vi "Configure Systems.vi"() -> ()   [LabVIEW 2009, in "POLARIS BME DG.lvlib" / "BME_DG_System.lvclass"]
doc: "Use this VI for creating a configuration file.\n\nUSAGE\n\n1. Detect all DGs. This action deaktivates all DGs. Make sure you plant will not be damage by this action.\n2. Create one or more systems by enter a systemname\n3. Add at leas one master and his slaves appropriate to Your HW configuration to system\n\n4. Switch to tab Define Cards. \n5. The array index is equal DGNr of DG. Name Your Cards an configure it\n6. Enter logical names for card channels\n\n7. Switch to tab Define Channels \n8. You can start by coping channel names from the card configuration\n9. Configure Your channels.\n\nTips:\nIf \"Error?\" is true some trouble inside delay formulas is detected. Pleace throw a glance into tab \"Check\", problem channels array may give You a hint.\nThe tab contains also a tool for calculation bit masks for \"Go Signal\" in channel configiration and for MS-Bus in cards configuration.\n\n---------------\n\nauthor: Alexander Kessler, Helmholtz-Institut-Jena \nmaintainer: Alexander Kessler: alexander.kessler@uni-jena.de\n\n\nLicense Agreement for this software:\n\nCopyright (C)\nHelmholtz-Institut-Jena\nFröbelsteg 3\n07743 Jena\nGermany\n\nContact: alexander.kessler@uni-jena.de\n\nThis program is free software; you can redistribute it and/or modify it under the terms of the GNU General Public License as published by the Free Software Foundation; either version 2 of the license, or (at your option) any later version.\n\nThis program is distributed in the hope that it will be useful, but WITHOUT ANY WARRANTY; without even the implied warranty of MERCHANTABILITY or FITNESS FOR A PARTICULAR PURPOSE. See the GNU General License for more details (http://www.gnu.org)."
uses:
  BME_DG_System.lvclass
  LV-BME Interface/DetectDG.ctl
  LV-BME Interface/System DG Selection.ctl
  LV-BME Interface/BME_DG_TriggerSettings.ctl
  LV-BME Interface/ClockSource.ctl
  LV-BME Interface/SG08_Settings.ctl
  LV-BME Interface/BME_DG_V2TriggerSettings.ctl
  LV-BME Interface/MSBusSignals.ctl
  LV-BME Interface/ChnlSettings.ctl
  LV-BME Interface/Go_Done_Chnl_Settings.ctl
  LV-BME Interface/GoSignalBits.ctl
  LV-BME Interface/SG08_Chnl_Settings.ctl
  LV-BME Interface/Chnl Settings Complete.ctl
  LV-BME Interface/Card Config.ctl
  BME_DG_Chnl/BME_DG_Chnl.lvclass
  POLARIS BME DG.lvlib
panel:
  out "Error?":bool
  in  "Build System":bool
  in  "ChnlToSwap":u16(ring) items=["a", "b", "c", "d", "e", "f", "ma", "mb", "mc", "md", "me", "mf", "sa", "sb", "sc", "sd", "se", "sf"]
  in  "SwapChnlWith":bool
  in  "Card2":u16(ring) caption="Swap with" items=["Master", "Master of Slave", "Slave of Master"]
  in  "SwapCardsWith":bool
  in  "Stop search":bool=TRUE
  in  "Find Chnl":u16(ring) items=["a", "b", "c", "d", "e", "f", "ma", "mb", "mc", "md", "me", "mf", "sa", "sb", "sc", "sd", "se", "sf"]
  in  "Find Card":u16(ring) items=["Master", "Master of Slave", "Slave of Master"]
  in  "stop":bool
  in  "Tab Control":T1(tab)=enum."Check"
  in  "InstalledDGs":T2[](array[typedef])
  in  "Select System":u16(ring) items=["Einsamer Master", "Master and Servant"]
  in  "Systems":T3[](array[typedef])
  in  "Selected DG":u16(ring) items=["0", "1", "2"]
  in  "Add":bool
  in  "Remove":bool
  in  "Empty Systems":bool
  in  "DetectDGs":bool
  in  "Card Config":T9(array[cluster]) {"Advanced Settings"."Trigger on MS Bus" format="%04x" items=["Local Primary0x1"=1, "Local Secondary0x2"=2, "Local Force 0x4"=4, "Resynchronize 0x8"=8, "StepBackOnBus 0x10"=16, "StartOnBus 0x20"=32, "InhibitOnBus 0x40"=64, "LoadDataOnBus 0x80"=128]; "Advanced Settings"."Force Trigger (µs)" min=0.0 format="%.6f"; "SG08_Settings"."StepBackTime (µs)" min=0.0 format="%.6f"; "SG08_Settings"."Gate Delay (µs)" format="%.3f"; "SG08_Settings"."Gate Level" min=-2.5 max=2.5 format="%.3g"; "Base Settings"."Gate Divider" min=1 max=1000000; "Base Settings"."Clock Source" items=["Internal Oscillator"=1, "External Trigger"=2, "Trigger-> Oscillator"=3, "MasterSlave Bus"=4]; "Base Settings"."Inhibit(µs)" format="%#_11g"}
  in  "Copy Chnl\n Names":bool=TRUE
  in  "Chnls":T14(array[cluster]) {"ChnParameter"."Delay (µs)" min=0.0 max=100000000.0 format="%.4f"; "G08_Chnl_Settings"."Pulse Width (µs)" min=0.0 max=8947840.0 format="%#.6f"; "Go and Done Signal"."Done Signal" format="%04x" items=["Local Primary"=1, "Local Secondary"=2, "Local Force"=4, "Master Primary"=16]; "Go and Done Signal"."Go Signal" format="%04x" items=["Local Primary0x1"=1, "Local Secondary0x2"=2, "Local Force 0x4"=4, "Resynchronize 0x8"=8, "Master Prim. 0x10"=16, "Master Sec. 0x20"=32, "Master Force  0x40"=64, "System Clock 0x80"=128, "Delay Clock 0x100"=256, "Inhibit Local 0x200"=512, "Start Local 0x400"=1024, "Start Bus 0x800"=2048, "Step Back Local 0x1000"=4096, "Step Back Bus 0x2000"=8192, "RunCircle 0x4000"=16384, "SyncReload 0x8000"=32768, "From E 0x10000"=65536, "From F 0x20000"=131072, "From Bus 0x40000"=262144]}
  in  "MS Signals Mask":u32 caption="Mask" format="%.0x"
  in  "MS Signals Bits to Mask":T8[](array[typedef]) format="%04x" items=["Local Primary0x1"=1, "Local Secondary0x2"=2, "Local Force 0x4"=4, "Resynchronize 0x8"=8, "StepBackOnBus 0x10"=16, "StartOnBus 0x20"=32, "InhibitOnBus 0x40"=64, "LoadDataOnBus 0x80"=128]
  in  "GoSignal Bits to Mask":T12[](array[typedef]) format="%04x" items=["Local Primary0x1"=1, "Local Secondary0x2"=2, "Local Force 0x4"=4, "Resynchronize 0x8"=8, "Master Prim. 0x10"=16, "Master Sec. 0x20"=32, "Master Force  0x40"=64, "System Clock 0x80"=128, "Delay Clock 0x100"=256, "Inhibit Local 0x200"=512, "Start Local 0x400"=1024, "Start Bus 0x800"=2048, "Step Back Local 0x1000"=4096, "Step Back Bus 0x2000"=8192, "RunCircle 0x4000"=16384, "SyncReload 0x8000"=32768, "From E 0x10000"=65536, "From F 0x20000"=131072, "From Bus 0x40000"=262144]
  in  "GoSignal Mask":u32 caption="Mask" format="%.0x"
  out "Problem Chnls out":string[](array[string])
  out "err and warnings":errorcluster[](array[cluster])
  out "Last Change":timestamp=timestamp(3422440183.453125 s since 1904-01-01)
  in  "Save":bool
  in  "Load":bool=TRUE
  in  "Config File":path
  # "DGNr"
  # "<=>"
  # "<=>"
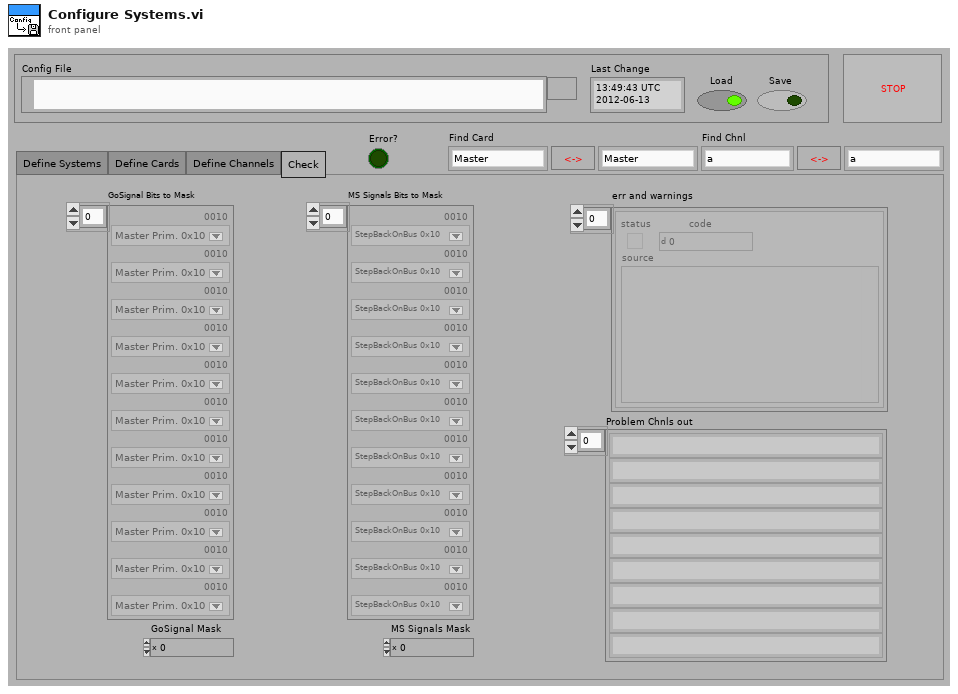
[diagram p1: front panel]
types:
  T1 = enum32{"Define Systems", "Define Cards", "Define Channels", "Check"}
  T2 = typedef "POLARIS BME DG.lvlib/DetectDG.ctl" = cluster{"DG_Number":i32, "DG_Product":i32, "Product Name":string, "Bus_Number":i32, "Slot_Number":i32, "Master":bool}
  T3 = typedef "POLARIS BME DG.lvlib/System DG Selection.ctl" = cluster{"Selected System DGs":T2[], "Name":string}
  T4 = typedef "POLARIS BME DG.lvlib/BME_DG_TriggerSettings.ctl" = cluster{"Clock Source":T5, " clock modulo":u32, "TriggerEnabled?":bool, "trigger modulo ":i32, "InputTerminated?":bool, "Inhibit(µs)":dbl, "TriggerLevel":dbl, "PresetValue":i32, "InternalTrigger?":bool, "InternalArm?":bool, "SWTrigger?":bool, "RisingEdge?":bool, "StopOnPreset?":bool, "ResetWhenDone?":bool, "Gate Divider":i32, "PositiveGate?":bool}
  T5 = typedef "POLARIS BME DG.lvlib/ClockSource.ctl" = i32
  T6 = typedef "POLARIS BME DG.lvlib/SG08_Settings.ctl" = cluster{"Gate Terminate":bool, "Gate Level":dbl, "Gate Delay (µs)":dbl, "StepBackTime (µs)":dbl, "Burst Counter":u32, "Trigger Divider":u32, "Trigger Multiplier":u32}
  T7 = typedef "POLARIS BME DG.lvlib/BME_DG_V2TriggerSettings.ctl" = cluster{"Trigger on MS Bus":T8, "Force Trigger (µs)":dbl, "Gate Type":bool, "Synchronize Gate":bool}
  T8 = typedef "POLARIS BME DG.lvlib/MSBusSignals.ctl" = u32
  T9 = cluster{"Logical Name":string, "Base Settings":T4, "SG08_Settings":T6, "Channel Names":string[], "Advanced Settings":T7}[]
  T10 = typedef "POLARIS BME DG.lvlib/ChnlSettings.ctl" = cluster{" Delay (µs)":dbl, "On?":bool, "PositiveVoltage?":bool, "50OhmTerminated? ":bool, "25OhmOutput?":bool}
  T11 = typedef "POLARIS BME DG.lvlib/Go_Done_Chnl_Settings.ctl" = cluster{"Go Signal":T12, "Done Signal":u32}
  T12 = typedef "POLARIS BME DG.lvlib/GoSignalBits.ctl" = u32
  T13 = typedef "POLARIS BME DG.lvlib/SG08_Chnl_Settings.ctl" = cluster{"Pulse Width (µs)":dbl, "Output Offset":u32, "Disconnect (E,F)":bool, "Onto MsBus (E,F)":bool, "Input Positive (E,F)":bool}
  T14 = cluster{"Channel Name":string, "ChnParameter":T10, "DelayFormula":string, "OutputModulo":i32, "Go and Done Signal":T11, "G08_Chnl_Settings":T13}[]
  T15 = typedef "POLARIS BME DG.lvlib/Chnl Settings Complete.ctl" = cluster{"Channel Name":string, "ChnParameter":T10, "DelayFormula":string, "OutputModulo":i32, "Go and Done Signal":T11, "G08_Chnl_Settings":T13}
  T16 = typedef "POLARIS BME DG.lvlib/Card Config.ctl" = cluster{"Logical Name":string, "Base Settings":T4, "SG08_Settings":T6, "Channel Names":string[], "Advanced Settings":T7}
  T17 = enum16{"open", "replace", "create", "open or create", "replace or create", "replace or create with confirmation"}
  T18 = cluster{"Logical Name":string, "Base Settings":T4, "SG08_Settings":T6, "Channel Names":string[], "Advanced Settings":T7}
  T19 = cluster{"Channel Name":string, "ChnParameter":T10, "DelayFormula":string, "OutputModulo":i32, "Go and Done Signal":T11, "G08_Chnl_Settings":T13}
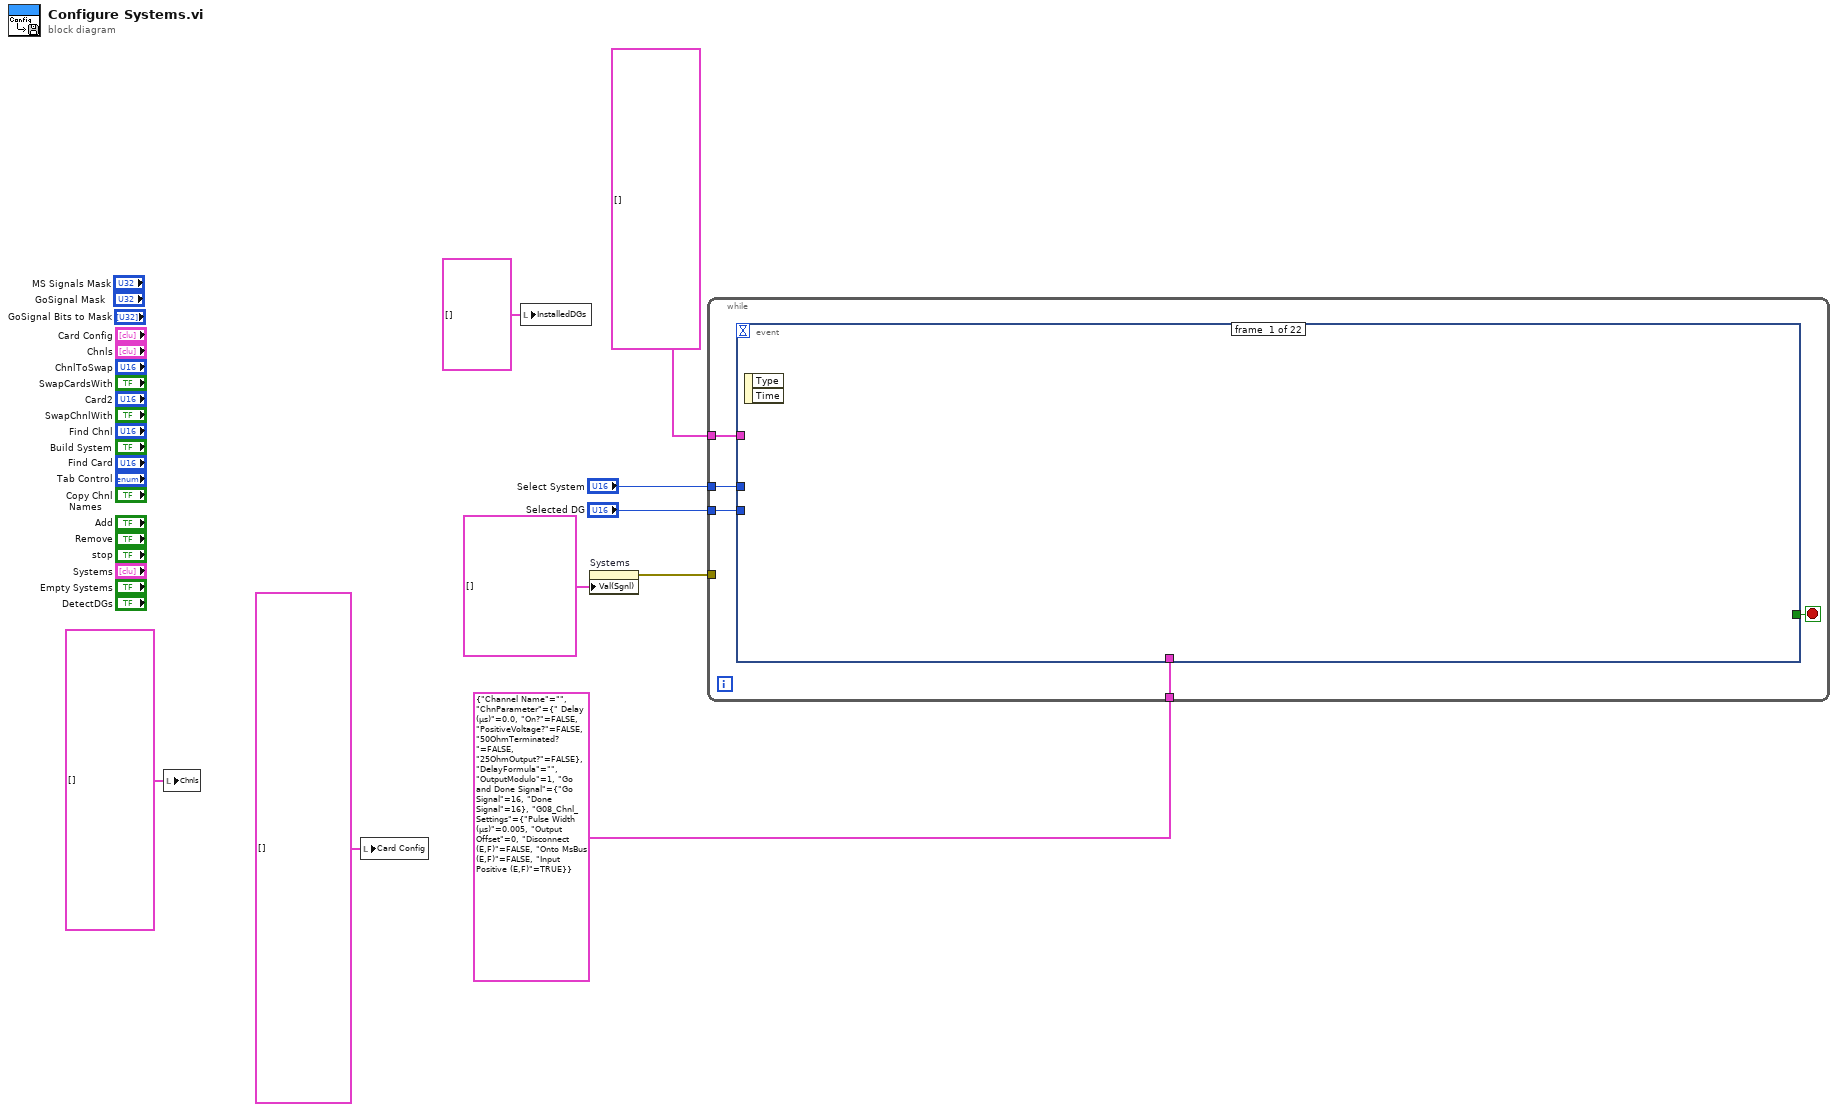
[diagram p0: block diagram]
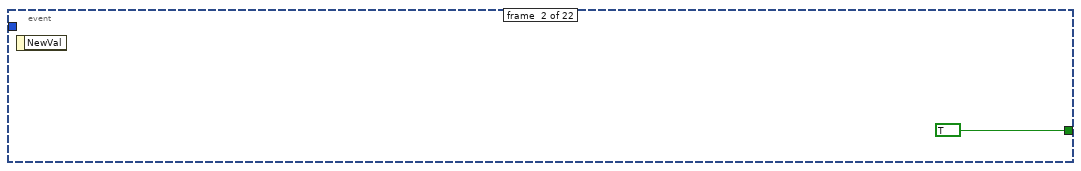
[diagram p2: hidden frame]
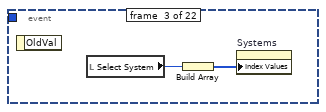
[diagram p3: hidden frame]
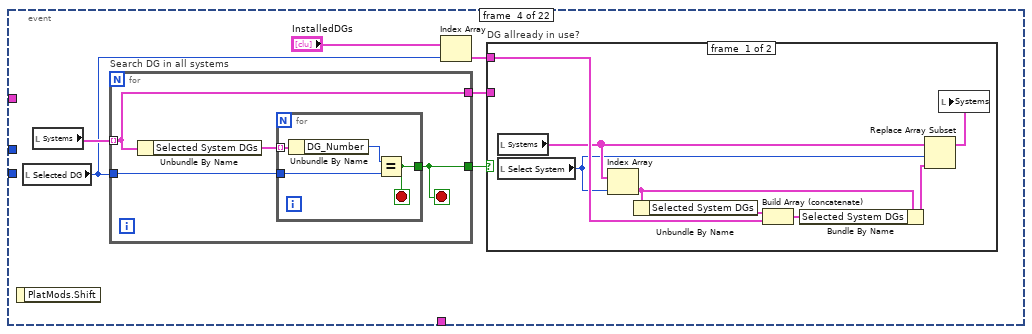
[diagram p4: hidden frame]
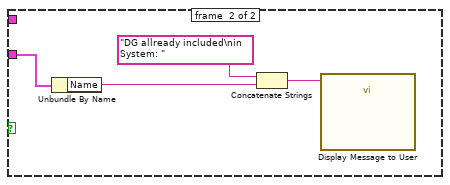
[diagram p5: hidden frame]
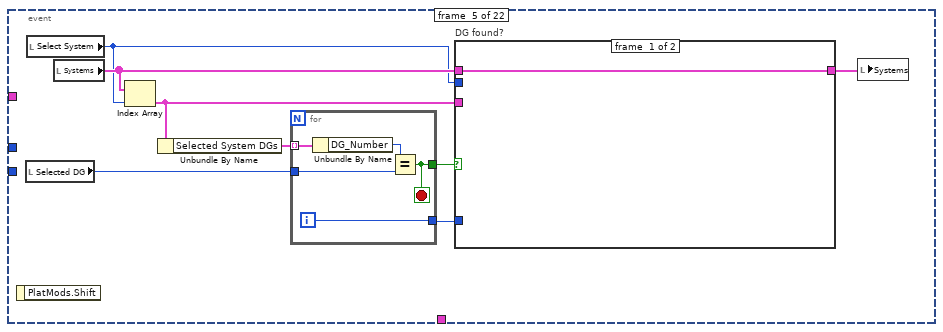
[diagram p6: hidden frame]
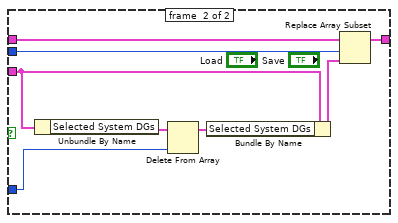
[diagram p7: hidden frame]
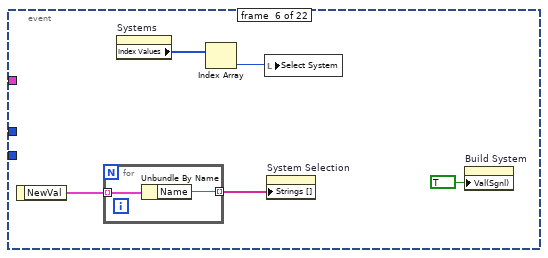
[diagram p8: hidden frame]
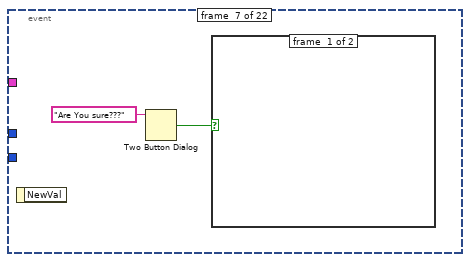
[diagram p9: hidden frame]
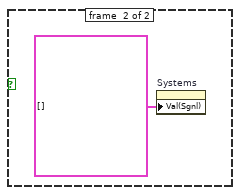
[diagram p10: hidden frame]
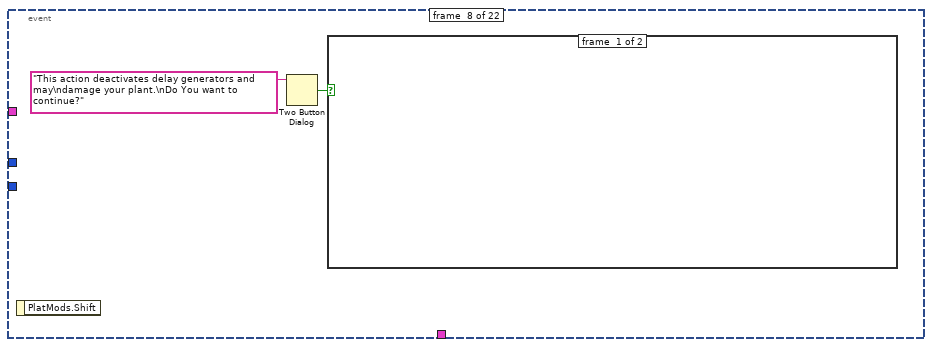
[diagram p11: hidden frame]
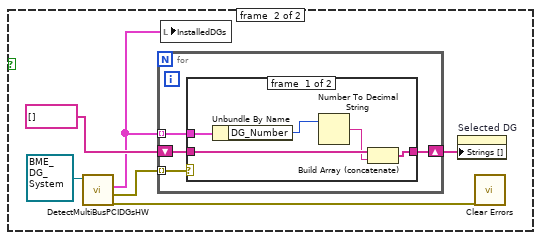
[diagram p12: hidden frame]
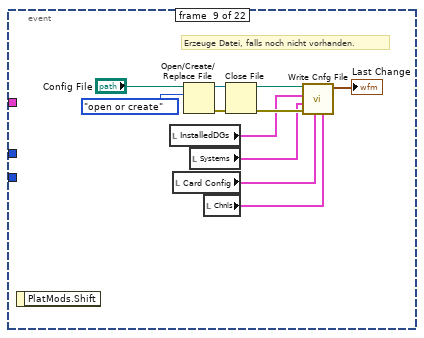
[diagram p14: hidden frame]
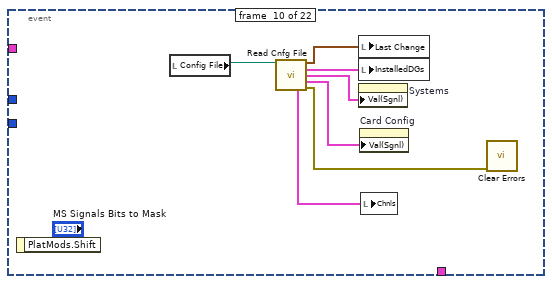
[diagram p15: hidden frame]
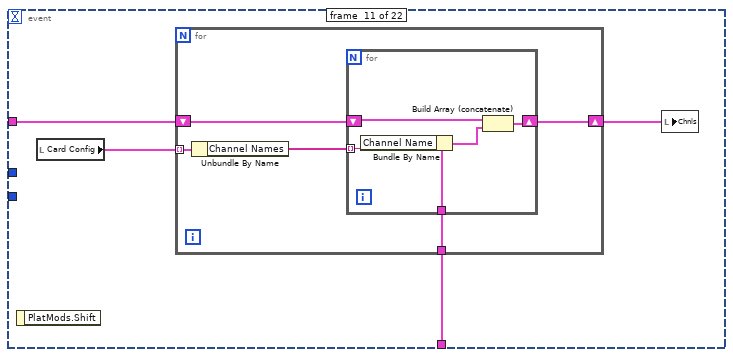
[diagram p16: hidden frame]
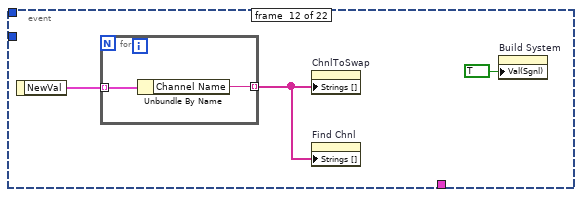
[diagram p17: hidden frame]
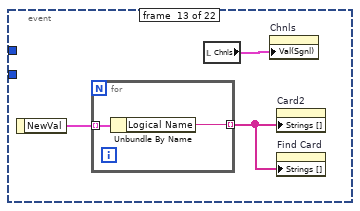
[diagram p18: hidden frame]
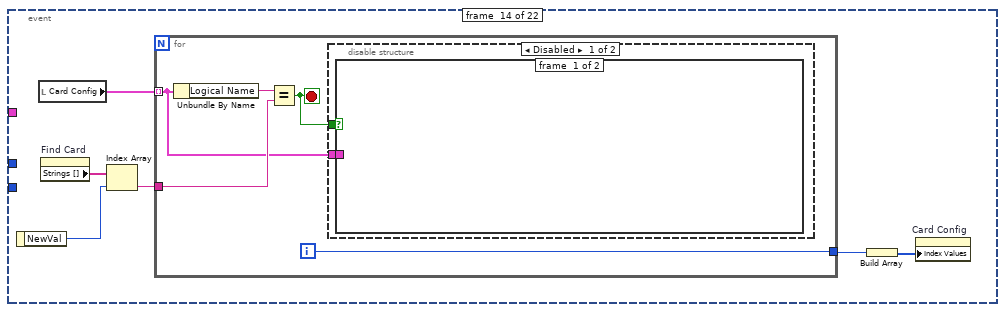
[diagram p19: hidden frame]
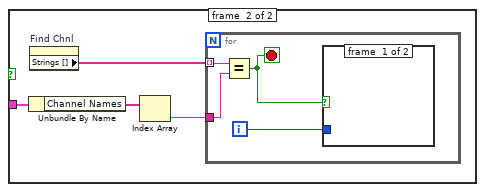
[diagram p20: hidden frame]
diagram:
  n1 = local write "Chnls"(T15[] [] ("Chnls")) -> ()
  n2 = local write "Card Config"(T16[] [] ("Card Config")) -> ()
  n3 = local write "InstalledDGs"(T2[] [] ("InstalledDGs")) -> ()
  n4 = property on="Systems" class="Arr (strict)"("Val(Sgnl)"=T3[] [] ("Value (Signaling)")) -> (error out=w6:errorcluster)  [unwired: 2 in, 1 out]
  n5 = while {
    tunnel: "Select System" -> [w13]
    tunnel: "Selected DG" -> [w12]
    tunnel: w6 -> [_]
    tunnel: T15 {"Channel Name"="", "ChnParameter"={" Delay (µs)"=0.0, "On?"=FALSE, "PositiveVoltage?"=FALSE, "50OhmTerminated? "=FALSE, "25OhmOutput?"=FALSE}, "DelayFormula"="", "OutputModulo"=1, "Go and Done Signal"={"Go Signal"=16, "Done Signal"=16}, "G08_Chnl_Settings"={"Pulse Width (µs)"=0.005, "Output Offset"=0, "Disconnect (E,F)"=FALSE, "Onto MsBus (E,F)"=FALSE, "Input Positive (E,F)"=TRUE}} ("Cluster") -> [w11]
    tunnel: T15[] [] -> [w10]
    stop <- w14 stop-if-true
    n6 = event shown="[8] \"Save\": Mouse Down;  \"Save\": Key Down" {
      selector: _ -> [_ _ _ _ _ _ _ _ _ _ _ _ _ _ _ _ _ _ _ _ _ _]
      dyn-events: _ -> [_ _ _ _ _ _ _ _ _ _ _ _ _ _ _ _ _ _ _ _ _ _]
      timeout: _ -> [_ _ _ _ _ _ _ _ _ _ _ _ _ _ _ _ _ _ _ _ _ _]
      tunnel: [_ TRUE _ _ _ _ _ _ _ _ _ _ _ _ _ _ _ _ _ _ _ _] -> w14
      tunnel: w13 -> [_ _ _ _ _ _ _ _ _ _ _ _ _ _ _ _ _ _ _ _ _ _]
      tunnel: w12 -> [_ _ _ _ _ _ _ _ _ _ _ _ _ _ _ _ _ _ _ _ _ _]
      tunnel: w11 -> [_ _ _ _ _ _ _ _ _ _ w113 _ _ _ _ _ _ _ _ _ _ _]
      tunnel: w10 -> [_ _ _ _ _ _ _ _ _ _ w112 _ _ _ _ _ _ _ _ _ _ _]
      event #0 {
        n7 = event-data() -> ()  [unwired: 1 in, 2 out]
      }
      event #1 {
        n8 = event-data() -> ()  [unwired: 1 in, 1 out]
      }
      event #2 {
        n9 = event-data() -> ()  [unwired: 1 in, 1 out]
        n10 = local read "Select System"() -> (w17:u16)
        n11 = Build Array(w17) -> (w16:u16[])
        n12 = property on="Systems" class="Arr (strict)"("Index Values"=w16) -> ()  [unwired: 2 in, 2 out]
      }
      event #3 {
        n13 = event-data() -> ()  [unwired: 1 in, 1 out]
        n14 = local read "Selected DG"() -> (w20:u16)
        n15 = local read "Systems"() -> (w23:T3[])
        n16 = for "Search DG in all systems" {
          tunnel: w23 -> [w36] mode=indexing
          tunnel: w20 -> [w38]
          tunnel: [w36] -> w21
          tunnel: [w37] -> w22
          stop <- w37 stop-if-true
          n17 = Unbundle By Name(w36) -> ("Selected System DGs"=w39:T2[])
          n18 = for {
            tunnel: w39 -> [w43] mode=indexing
            tunnel: w38 -> [w42]
            tunnel: [w40] -> w37
            stop <- w40 stop-if-true
            n19 = Unbundle By Name(w43) -> ("DG_Number"=w41:i32)
            n20 = Equal?(x=w41, y=w42) -> (x = y?=w40:bool)
          }
        }
        n21 = Index Array(array="InstalledDGs", index=w20) -> (element=w19:T2)
        n22 = case "DG allready in use?" shown="False" w22 {
          tunnel: w21 -> [_ w35]
          tunnel: w19 -> [w29 _]
          frame #0 {
            n23 = local read "Systems"() -> (w26:T3[])
            n24 = local read "Select System"() -> (w25:u16)
            n25 = Index Array(array=w26, index=w25) -> (element=w24:T3)
            n26 = Unbundle By Name(w24) -> ("Selected System DGs"=w31:T2[])
            n27 = Build Array (concatenate)(w31, w29) -> (w30:T2[])
            n28 = Bundle By Name(cluster=w24, "Selected System DGs"=w30) -> (w27:T3)
            n29 = Replace Array Subset(array=w26, new element=w27, index=w25) -> (w28:T3[])
            n30 = local write "Systems"(w28) -> ()
          }
          frame #1 {
            n31 = Unbundle By Name(w35) -> ("Name"=w32:string)
            n32 = Concatenate Strings("DG allready included\nin System: " ("string"), w32) -> (w34:string)
            n33 = call "Display Message to User"("Message"=w34) -> ()  [unwired: 9 in, 2 out]
          }
        }
      }
      event #4 {
        n34 = event-data() -> ()  [unwired: 1 in, 1 out]
        n35 = local read "Selected DG"() -> (w47:u16)
        n36 = local read "Select System"() -> (w44:u16)
        n37 = local read "Systems"() -> (w48:T3[])
        n38 = Index Array(array=w48, index=w44) -> (element=w45:T3)
        n39 = Unbundle By Name(w45) -> ("Selected System DGs"=w46:T2[])
        n40 = for {
          tunnel: w46 -> [w52] mode=indexing
          tunnel: w47 -> [w56]
          tunnel: [w55] -> w51
          tunnel: [w54] -> w50
          i -> [w54]
          stop <- w55 stop-if-true
          n41 = Unbundle By Name(w52) -> ("DG_Number"=w53:i32)
          n42 = Equal?(x=w53, y=w56) -> (x = y?=w55:bool)
        }
        n43 = case "DG found?" shown="True" w51 {
          tunnel: w50 -> [_ w62]
          tunnel: w48 -> [w57 w65]
          tunnel: [w57 w64] -> w49
          tunnel: w45 -> [_ w61]
          tunnel: w44 -> [_ w58]
          frame #0 {
          }
          frame #1 {
            n44 = Unbundle By Name(w61) -> ("Selected System DGs"=w63:T2[])
            n45 = Delete From Array(array=w63, index=w62) -> (array with subset deleted=w60:T2[])  [unwired: 1 in, 1 out]
            n46 = Bundle By Name(cluster=w61, "Selected System DGs"=w60) -> (w59:T3)
            n47 = Replace Array Subset(array=w65, new element=w59, index=w58) -> (w64:T3[])
          }
        }
        n48 = local write "Systems"(w49) -> ()
      }
      event #5 {
        n49 = event-data() -> ("NewVal"=w70:T3[])  [unwired: 1 in]
        n50 = for {
          tunnel: w70 -> [w72] mode=indexing
          tunnel: [w71] -> w69 mode=indexing
          n51 = Unbundle By Name(w72) -> ("Name"=w71:string)
        }
        n52 = property on="Systems" class="Arr (strict)"() -> ("Index Values"=w68:u32[])  [unwired: 2 in, 2 out]
        n53 = Index Array(array=w68) -> (element=w67:u32)  [unwired: 1 in]
        n54 = local write "Select System"(w67) -> ()
        n55 = property on="System Selection" class="Ring (strict)"("Strings []"=w69) -> ()  [unwired: 2 in, 2 out]
        n56 = property on="Build System" class="Bool (strict)"("Val(Sgnl)"=TRUE ("Value (Signaling)")) -> ()  [unwired: 2 in, 2 out]
      }
      event #6 {
        n57 = event-data() -> ()  [unwired: 1 in, 1 out]
        n58 = Two Button Dialog(message="Are You sure???") -> (T button?=w73:bool)  [unwired: 2 in]
        n59 = case shown="True" w73 {
          frame #0 {
          }
          frame #1 {
            n60 = property on="Systems" class="Arr (strict)"("Val(Sgnl)"=T3[] [] ("Value (Signaling)")) -> ()  [unwired: 2 in, 2 out]
          }
        }
      }
      event #7 {
        n61 = event-data() -> ()  [unwired: 1 in, 1 out]
        n62 = Two Button Dialog(message="This action deactivates delay generators and may\ndamage your plant.\nDo You want to continue?") -> (T button?=w76:bool)  [unwired: 2 in]
        n63 = case shown="True" w76 {
          frame #0 {
          }
          frame #1 {
            n64 = call "DetectMultiBusPCIDGsHW.vi"("BME_DG_System in"=refnum<class "BME_DG_System.lvclass"> refnum) -> ("error out"=w78:errorcluster, "Errors"=w81:errorcluster[], "InstalledDGs"=w79:T2[])  [unwired: 6 in, 2 out]
            n65 = for {
              tunnel: w81 -> [w84] mode=indexing
              tunnel: w79 -> [w86] mode=indexing
              shift-right: [w87] -> w82
              shift-left: string[] [] -> [w85]
              n66 = case shown="No Error" w84 {
                tunnel: [w92 w93] -> w87
                tunnel: w86 -> [w90 _]
                tunnel: w85 -> [w91 w93]
                frame #0 {
                  n67 = Unbundle By Name(w90) -> ("DG_Number"=w89:i32)
                  n68 = Number To Decimal String(number=w89) -> (decimal integer string=w88:string)  [unwired: 1 in]
                  n69 = Build Array (concatenate)(w91, w88) -> (w92:string[])
                }
                frame #1 {
                }
              }
            }
            n70 = local write "InstalledDGs"(w79) -> ()
            n71 = property on="Selected DG" class="Ring (strict)"("Strings []"=w82) -> ()  [unwired: 2 in, 2 out]
            n72 = call <vilib>:"Clear Errors.vi"("error in (no error)"=w78) -> ()  [unwired: 6 in, 1 out]
          }
        }
      }
      event #8 {
        # "Erzeuge Datei, falls noch nicht vorhanden."
        n73 = event-data() -> ()  [unwired: 1 in, 1 out]
        n74 = local read "InstalledDGs"() -> (w98:T2[])
        n75 = local read "Card Config"() -> (w96:T9)
        n76 = Open/Create/Replace File(file path (use dialog)="Config File", operation (0:open)=T17."open or create") -> (refnum out=w103:refnum<file>, error out=w102:errorcluster)  [unwired: 4 in, 1 out]
        n77 = local read "Systems"() -> (w97:T3[])
        n78 = local read "Chnls"() -> (w95:T14)
        n79 = Close File(refnum=w103, error in=w102) -> (path=w100:path, error out=w99:errorcluster)
        n80 = call "Write Cnfg File.vi"("Chnls"=w95, "Cards"=w96, "error in"=w99, "DGSystems"=w97, "InstalledDGs"=w98, "pathConfigFile"=w100) -> ("current time"=→"Last Change":timestamp)  [unwired: 4 in, 1 out]
      }
      event #9 {
        n81 = event-data() -> ()  [unwired: 1 in, 1 out]
        n82 = local read "Config File"() -> (w111:path)
        n83 = call "Read Cnfg File.vi"("Config File"=w111) -> ("Last Change"=w110:timestamp, "InstalledDGs"=w109:T2[], "DGSystems"=w108:T3[], "Cards"=w107:T16[], "Chnls"=w106:T15[], "error out"=w105:errorcluster)  [unwired: 9 in]
        n84 = local write "Last Change"(w110) -> ()
        n85 = local write "InstalledDGs"(w109) -> ()
        n86 = property on="Systems" class="Arr (strict)"("Val(Sgnl)"=w108) -> ()  [unwired: 2 in, 2 out]
        n87 = property on="Card Config" class="Arr (strict)"("Val(Sgnl)"=w107) -> ()  [unwired: 2 in, 2 out]
        n88 = local write "Chnls"(w106) -> ()
        n89 = call <vilib>:"Clear Errors.vi"("error in (no error)"=w105) -> ()  [unwired: 6 in, 1 out]
      }
      event #10 {
        n90 = event-data() -> ()  [unwired: 1 in, 1 out]
        n91 = local read "Card Config"() -> (w115:T9)
        n92 = for {
          tunnel: w115 -> [w120] mode=indexing
          shift-right: [w117] -> w114
          shift-left: w112 -> [w118]
          tunnel: w113 -> [w116]
          n93 = Unbundle By Name(w120) -> ("Channel Names"=w119:string[])
          n94 = for {
            tunnel: w119 -> [w122] mode=indexing
            shift-right: [w124] -> w117
            shift-left: w118 -> [w125]
            tunnel: w116 -> [w123]
            n95 = Bundle By Name(cluster=w123, "Channel Name"=w122) -> (w121:T15)
            n96 = Build Array (concatenate)(w125, w121) -> (w124:T15[])
          }
        }
        n97 = local write "Chnls"(w114) -> ()
      }
      event #11 {
        n98 = event-data() -> ("NewVal"=w128:T14)  [unwired: 1 in]
        n99 = for {
          tunnel: w128 -> [w129] mode=indexing
          tunnel: [w130] -> w127 mode=indexing
          n100 = Unbundle By Name(w129) -> ("Channel Name"=w130:string)
        }
        n101 = property on="ChnlToSwap" class="Ring (strict)"("Strings []"=w127) -> ()  [unwired: 2 in, 2 out]
        n102 = property on="Find Chnl" class="Ring (strict)"("Strings []"=w127) -> ()  [unwired: 2 in, 2 out]
        n103 = property on="Build System" class="Bool (strict)"("Val(Sgnl)"=TRUE ("Value (Signaling)")) -> ()  [unwired: 2 in, 2 out]
      }
      event #12 {
        n104 = event-data() -> ("NewVal"=w133:T9)  [unwired: 1 in]
        n105 = for {
          tunnel: w133 -> [w135] mode=indexing
          tunnel: [w134] -> w132 mode=indexing
          n106 = Unbundle By Name(w135) -> ("Logical Name"=w134:string)
        }
        n107 = local read "Chnls"() -> (w131:T14)
        n108 = property on="Chnls" class="Arr (strict)"("Val(Sgnl)"=w131) -> ()  [unwired: 2 in, 2 out]
        n109 = property on="Card2" class="Ring (strict)"("Strings []"=w132) -> ()  [unwired: 2 in, 2 out]
        n110 = property on="Find Card" class="Ring (strict)"("Strings []"=w132) -> ()  [unwired: 2 in, 2 out]
      }
      event #13 {
        n111 = event-data() -> ("NewVal"=w137:u16)  [unwired: 1 in]
        n112 = local read "Card Config"() -> (w139:T9)
        n113 = property on="Find Card" class="Ring (strict)"() -> ("Strings []"=w138:string[])  [unwired: 2 in, 2 out]
        n114 = Index Array(array=w138, index=w137) -> (element=w140:string)
        n115 = for {
          tunnel: w139 -> [w142] mode=indexing
          tunnel: w140 -> [w145]
          tunnel: [w144] -> w141
          i -> [w144]
          stop <- w143 stop-if-true
          n116 = Unbundle By Name(w142) -> ("Logical Name"=w146:string)
          n117 = Equal?(x=w146, y=w145) -> (x = y?=w143:bool)
          n118 = disable-structure shown="Disabled" {
            disable-tunnel: w143 -> [w148 _]
            disable-tunnel: w142 -> [w147 _]
            frame #0 {
              n119 = case shown="True" w148 {
                tunnel: w147 -> [_ w151]
                frame #0 {
                }
                frame #1 {
                  n120 = Unbundle By Name(w151) -> ("Channel Names"=w150:string[])
                  n121 = property on="Find Chnl" class="Ring (strict)"() -> ("Strings []"=w152:string[])  [unwired: 2 in, 2 out]
                  n122 = Index Array(array=w150) -> (element=w149:string)  [unwired: 1 in]
                  n123 = for {
                    tunnel: w152 -> [w156] mode=indexing
                    tunnel: w149 -> [w155]
                    i -> [w153]
                    stop <- w154 stop-if-true
                    n124 = Equal?(x=w156, y=w155) -> (x = y?=w154:bool)
                    n125 = case shown="True" w154 {
                      selector: w154 -> [_ w157]
                      tunnel: w153 -> [_ w158]
                      frame #0 {
                      }
                      frame #1 {
                        n126 = local write "Stop search"(w157) -> ()
                        n127 = property on="Find Chnl" class="Ring (strict)"("Val(Sgnl)"=w158) -> ()  [unwired: 2 in, 2 out]
                      }
                    }
                  }
                }
              }
            }
            frame #1 {
            }
          }
        }
        n128 = Build Array(w141) -> (w136:i32[])
        n129 = property on="Card Config" class="Arr (strict)"("Index Values"=w136) -> ()  [unwired: 2 in, 2 out]
      }
      event #14 {
        n130 = event-data() -> ("NewVal"=w169:u16)  [unwired: 1 in]
        n131 = local read "Card Config"() -> (w170:T9)
        n132 = property on="Find Chnl" class="Ring (strict)"() -> ("Strings []"=w168:string[])  [unwired: 2 in, 2 out]
        n133 = Index Array(array=w168, index=w169) -> (element=w163:string)
        n134 = for {
          tunnel: w170 -> [w184] mode=indexing
          tunnel: w163 -> [w182]
          tunnel: [w181] -> w167
          tunnel: [w180] -> w166
          i -> [w181]
          stop <- w180 stop-if-true
          n135 = Unbundle By Name(w184) -> ("Channel Names"=w183:string[])
          n136 = for {
            tunnel: w183 -> [w186] mode=indexing
            tunnel: w182 -> [w187]
            tunnel: [w185] -> w180
            stop <- w185 stop-if-true
            n137 = Equal?(x=w186, y=w187) -> (x = y?=w185:bool)
          }
        }
        n138 = Not(x="Stop search") -> (.not. x?=w159:bool)
        n139 = And(x=w166, y=w159) -> (x .and. y?=w161:bool)
        n140 = local read "Chnls"() -> (w165:T14)
        n141 = case shown="True" w161 {
          tunnel: w167 -> [_ w179]
          frame #0 {
            n142 = local write "Stop search"(FALSE ("Stop search")) -> ()
          }
          frame #1 {
            n143 = property on="Find Card" class="Ring (strict)"("Val(Sgnl)"=w179) -> ()  [unwired: 2 in, 2 out]
          }
        }
        n144 = for {
          tunnel: w165 -> [w177] mode=indexing
          tunnel: w163 -> [w175]
          tunnel: [w174] -> w164
          tunnel: [w173] -> w162
          i -> [w174]
          stop <- w173 stop-if-true
          n145 = Unbundle By Name(w177) -> ("Channel Name"=w176:string)
          n146 = Equal?(x=w175, y=w176) -> (x = y?=w173:bool)
        }
        n147 = case shown="True" w162 {
          tunnel: w164 -> [_ w171]
          frame #0 {
          }
          frame #1 {
            n148 = Build Array(w171) -> (w172:i32[])
            n149 = property on="Chnls" class="Arr (strict)"("Index Values"=w172) -> ()  [unwired: 2 in, 2 out]
          }
        }
      }
      event #15 {
        n150 = event-data() -> ("NewVal"=w190:T12[])  [unwired: 1 in]
        n151 = for {
          tunnel: w190 -> [w193] mode=indexing
          shift-right: [w192] -> w188
          shift-left: 0 -> [w191]
          n152 = Or(x=w191, y=w193) -> (x .or. y?=w192:T12)
        }
        n153 = local write "GoSignal Mask"(w188) -> ()
      }
      event #16 {
        n154 = event-data() -> ("NewVal"=w196:T8[])  [unwired: 1 in]
        n155 = for {
          tunnel: w196 -> [w199] mode=indexing
          shift-right: [w198] -> w194
          shift-left: 0 -> [w197]
          n156 = Or(x=w197, y=w199) -> (x .or. y?=w198:T8)
        }
        n157 = local write "MS Signals Mask"(w194) -> ()
      }
      event #17 {
        n158 = event-data() -> ("NewVal"=w200:bool)  [unwired: 1 in]
        n159 = case shown="True" w200 {
          frame #0 {
          }
          frame #1 {
            n160 = local read "Card Config"() -> (w207:T9)
            n161 = local read "Find Card"() -> (w205:u16)
            n162 = local read "Card2"() -> (w202:u16)
            n163 = Index Array(array=w207, index #1=w205, index #2=w202) -> (element #1=w203:T18, element #2=w204:T18)
            n164 = Replace Array Subset(array=w207, new element=w204, index=w205) -> (w206:T9)
            n165 = Replace Array Subset(array=w206, new element=w203, index=w202) -> (w201:T9)
            n166 = property on="Card Config" class="Arr (strict)"("Val(Sgnl)"=w201) -> ()  [unwired: 2 in, 2 out]
          }
        }
      }
      event #18 {
        n167 = event-data() -> ()  [unwired: 1 in, 2 out]
        n168 = local read "Chnls"() -> (w210:T14)
        n169 = local read "Find Chnl"() -> (w209:u16)
        n170 = local read "ChnlToSwap"() -> (w208:u16)
        n171 = Index Array(array=w210, index #1=w209, index #2=w208) -> (element #1=w212:T19, element #2=w213:T19)
        n172 = Replace Array Subset(array=w210, new element=w213, index=w209) -> (w214:T14)
        n173 = Replace Array Subset(array=w214, new element=w212, index=w208) -> (w211:T14)
        n174 = property on="Chnls" class="Arr (strict)"("Val(Sgnl)"=w211) -> ()  [unwired: 2 in, 2 out]
      }
      event #19 {
        n175 = event-data() -> ("NewVal"=w218:u32)  [unwired: 1 in]
        n176 = Number To Boolean Array(number=w218) -> (Boolean array=w217:bool[])
        n177 = for {
          tunnel: w217 -> [w222] mode=indexing
          shift-right: [w219] -> w215
          shift-left: i32[] [] ("Array") -> [w220]
          i -> [w221]
          n178 = case shown="True" w222 {
            tunnel: w221 -> [_ w227]
            tunnel: w220 -> [w223 w225]
            tunnel: [w223 w224] -> w219
            frame #0 {
            }
            frame #1 {
              n179 = Logical Shift(y=w227, x=1) -> (x << y=w226:i32)
              n180 = Build Array (concatenate)(w225, w226) -> (w224:i32[])
            }
          }
        }
        n181 = local write "GoSignal Bits to Mask"(w215) -> ()
      }
      event #20 {
        n182 = event-data() -> ("NewVal"=w232:u32)  [unwired: 1 in]
        n183 = Number To Boolean Array(number=w232) -> (Boolean array=w231:bool[])
        n184 = for {
          tunnel: w231 -> [w236] mode=indexing
          shift-right: [w233] -> w229
          shift-left: i32[] [] ("Array") -> [w234]
          i -> [w235]
          n185 = case shown="True" w236 {
            tunnel: w235 -> [_ w241]
            tunnel: w234 -> [w237 w239]
            tunnel: [w237 w238] -> w233
            frame #0 {
            }
            frame #1 {
              n186 = Logical Shift(y=w241, x=1) -> (x << y=w240:i32)
              n187 = Build Array (concatenate)(w239, w240) -> (w238:i32[])
            }
          }
        }
        n188 = local write "MS Signals Bits to Mask"(w229) -> ()
      }
      event #21 {
        n189 = event-data() -> ("NewVal"=w243:bool)  [unwired: 1 in]
        n190 = case shown="True" w243 {
          frame #0 {
          }
          frame #1 {
            n191 = local read "Card Config"() -> (w255:T9)
            n192 = local read "Systems"() -> (w256:T3[])
            n193 = local read "Chnls"() -> (w251:T14)
            n194 = for {
              tunnel: [w279] -> w252 mode=indexing
              tunnel: [w278] -> w250
              tunnel: w256 -> [w277] mode=indexing
              tunnel: w255 -> [w276]
              tunnel: w251 -> [w275]
              tunnel: [w274] -> w246 mode=indexing
              tunnel: refnum<class "BME_DG_System.lvclass"> refnum ("BME_DG_System in") -> [w273]
              n195 = call "InitDGSystem and HW.vi"("InitHW(false)"=FALSE ("InitHW(True)"), "System"=w277, "Chnls"=w275, "Cards"=w276, "BME_DG_System in"=w273) -> ("error out"=w274:errorcluster, "Problem Chnls out"=w278:string[], "BME_DG_System in"=w279:refnum<class "BME_DG_System.lvclass">)  [unwired: 4 in]
            }
            n196 = for "Show Abs Delayvalues" {
              tunnel: w251 -> [w263] mode=indexing
              tunnel: [w261] -> w253 mode=indexing
              tunnel: w252 -> [w267]
              tunnel: [w260] -> w248 mode=indexing
              shift-right: [w258] -> w249
              shift-left: w250 -> [w259]
              n197 = Unbundle By Name(w263) -> ("Channel Name"=w257:string)
              n198 = call "Select System By Chnl.vi"("ChnlName"=w257, "SystemsIn"=w267) -> ("error out"=w266:errorcluster, "BME_DG_Chnl"=w265:refnum<class "BME_DG_Chnl.lvclass">)  [unwired: 5 in, 3 out]
              n199 = call-dynamic "Read ChnParameter.vi"("error in (no error)"=w266, "BME_DG_Chnl in"=w265) -> ("error out"=w260:errorcluster, "ChnParemater"=w264:T10)  [unwired: 4 in, 4 out]
              n200 = Unbundle By Name(w264) -> ("Delay (µs)"=w262:dbl)
              n201 = case shown="Error" w260 {
                tunnel: w259 -> [w268 w271]
                tunnel: [w268 w270] -> w258
                tunnel: w257 -> [_ w269]
                frame #0 {
                }
                frame #1 {
                  n202 = Build Array (concatenate)(w271, w269) -> (w270:string[])
                }
              }
              n203 = Bundle By Name(cluster=w263, "ChnParameter.Delay (µs)"=w262) -> (w261:T19)
            }
            "Problem Chnls out" <- w249
            n204 = local write "Chnls"(w253) -> ()
            n205 = Build Array (concatenate)(w248, w246) -> (w247:errorcluster[])
            n206 = call "Remove empty Errors.vi"("all error clusters"=w247) -> ("err and warnings"=→"err and warnings":errorcluster[], "some problems?"=→"Error?":bool)  [unwired: 9 in]
          }
        }
      }
    }
  }
